vi "statemachine.vi"() -> ()   [LabVIEW 2022 SP3]
uses:
  CV7/Control 1.ctl
panel:
  in  "Boolean":bool
  in  "stop":bool
  out "Enum 2":T1
  in  "Enum":T1
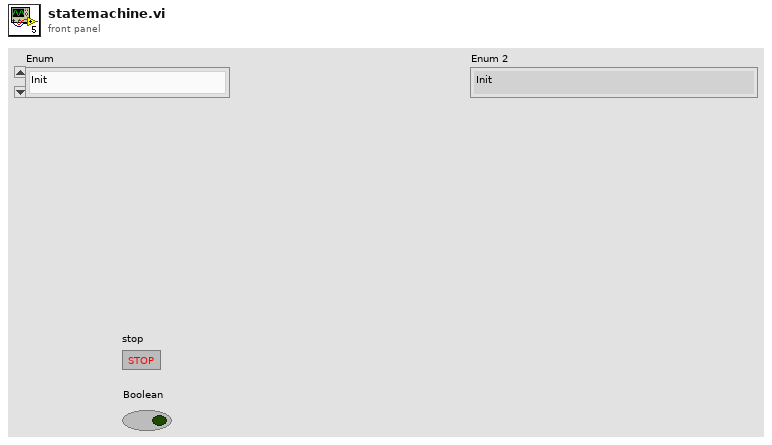
[diagram p1: front panel]
types:
  T1 = typedef "Control 1.ctl" = enum16{"Init\n", "Measure\n", "Wait\n", "End\n"}
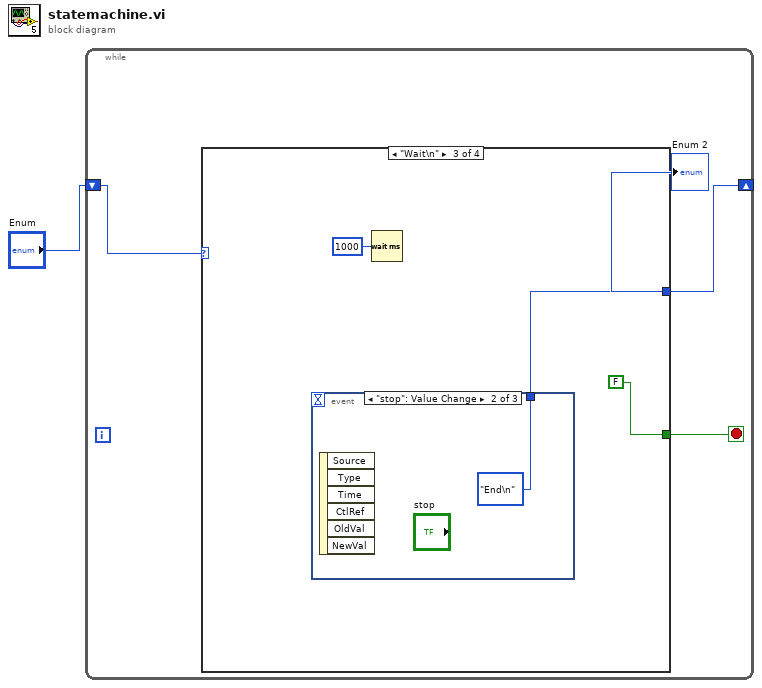
[diagram p0: block diagram]
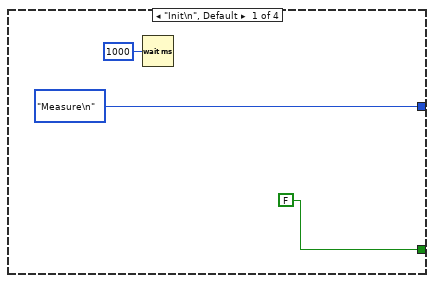
[diagram p2: hidden frame]
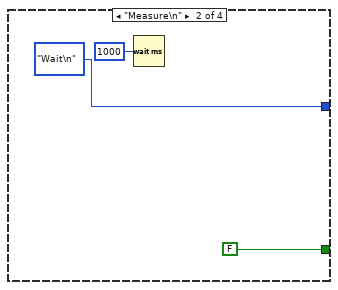
[diagram p3: hidden frame]
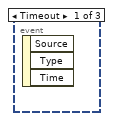
[diagram p4: hidden frame]
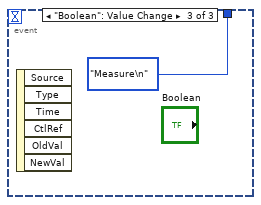
[diagram p5: hidden frame]
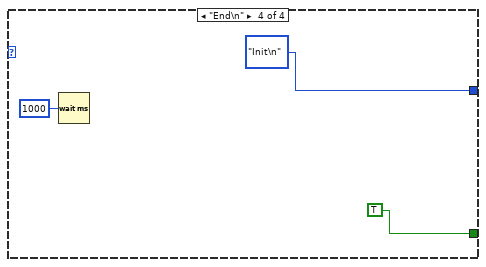
[diagram p6: hidden frame]
diagram:
  n1 = while {
    shift-right: [w3] -> _
    shift-left: "Enum" -> [w4]
    stop <- w2 stop-if-true
    n2 = case shown="\"Wait\\n\"" w4 {
      tunnel: [Control_1."Measure\n" ("Enum 2") Control_1."Wait\n" ("Enum 2") w12 Control_1."Init\n" ("Enum 2")] -> w3
      tunnel: [FALSE FALSE FALSE TRUE] -> w2
      frame "Init\n", Default {
        n3 = Wait (ms)(milliseconds to wait=u32 1000) -> ()  [unwired: 1 out]
      }
      frame "Measure\n" {
        n4 = Wait (ms)(milliseconds to wait=u32 1000) -> ()  [unwired: 1 out]
      }
      frame "Wait\n" {
        n5 = event shown="[1] \"stop\": Value Change" {
          selector: _ -> [_ _ _]
          dyn-events: _ -> [_ _ _]
          timeout: _ -> [_ _ _]
          tunnel: [_ Control_1."End\n" ("Enum 2") Control_1."Measure\n" ("Enum 2")] -> w12
          event Timeout {
            n6 = event-data() -> ()  [unwired: 1 in, 3 out]
          }
          event "stop": Value Change {
            n7 = event-data() -> ()  [unwired: 1 in, 6 out]
          }
          event "Boolean": Value Change {
            n8 = event-data() -> ()  [unwired: 1 in, 6 out]
          }
        }
        n9 = Wait (ms)(milliseconds to wait=u32 1000) -> ()  [unwired: 1 out]
      }
      frame "End\n" {
        n10 = Wait (ms)(milliseconds to wait=u32 1000) -> ()  [unwired: 1 out]
      }
    }
    "Enum 2" <- w3
  }
